vi "DIAdem Close.vi"(8 "error in (no error)":errorcluster, 10 "DD queue":T1, 11 "DIAdem Reference":T2) -> (0 "error out":errorcluster)   [LabVIEW 2011]
uses:
  <vilib>/ExportToExcel/DIAdem Reference.ctl
  DIAdem Queues.ctl
  DIAdem Daemon Queue.ctl
  DIAdem Daemon Script Type.ctl
  Datasheet/Datasheet Inputs.ctl
  www/cgi-bin/_cgi-lib/TDM_INDEX Record.ctl
  Datasheet/Datasheet Generator Settings.ctl
  www/cgi-bin/runtest/runtest Queue.ctl
  www/tests/Test Output.ctl
  database/Fields/Field Record.ctl
  database/Fields/Field DataTypes.ctl
  database/Fields/Field NextItem.ctl
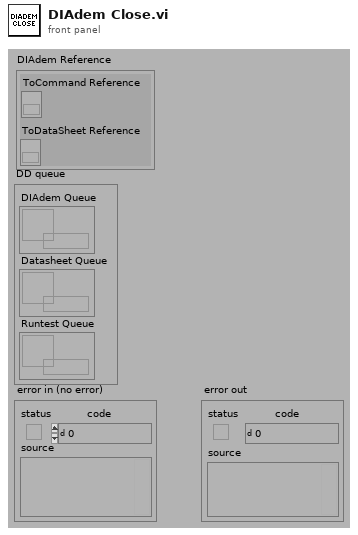
[diagram p1: front panel]
types:
  T1 = typedef "DIAdem Queues.ctl" = cluster{"DIAdem Queue":refnum<queue>, "Datasheet Queue":refnum<queue>, "Runtest Queue":refnum<queue>}
  T2 = typedef "DIAdem Reference.ctl" = cluster{"ToCommand Reference":refnum<k7>, "ToDataSheet Reference":refnum<k7>}
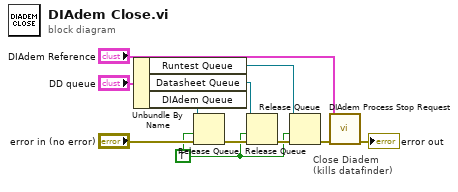
[diagram p0: block diagram]
diagram:
  w1 = TRUE
  # "Close Diadem\n(kills datafinder)"
  n1 = Unbundle By Name("DD queue") -> ("Runtest Queue"=w2:refnum<queue>, "Datasheet Queue"=w3:refnum<queue>, "DIAdem Queue"=w4:refnum<queue>)
  n2 = Release Queue(queue=w4, force destroy? (F)=w1, error in (no error)="error in (no error)") -> (error out=w5:errorcluster)  [unwired: 2 out]
  n3 = Release Queue(queue=w3, force destroy? (F)=w1, error in (no error)=w5) -> (error out=w6:errorcluster)  [unwired: 2 out]
  n4 = Release Queue(queue=w2, force destroy? (F)=w1, error in (no error)=w6) -> (error out=w7:errorcluster)  [unwired: 2 out]
  n5 = call "DIAdem Process Stop Request.vi"("error in (no error)"=w7, "DIAdem Reference"="DIAdem Reference") -> ("error out"=→"error out":errorcluster)  [unwired: 4 in, 2 out]
